vi "UDP Data Link - Configuration Utilities - Update Properties.vi"(6 "Tx?":bool, 8 "error in (no error)":errorcluster, 9 "Channel Paths":string[](array[string]), 10 "Channel Names":string[](array[string]), 11 "Item Ref in":T1 format="%.0x") -> (0 "error out":errorcluster, 3 "Item Ref out":T1=18446744073709551615 format="%.0x")   [LabVIEW 2015, in "UDP-Custom-Device System Explorer.lvlib"]
uses:
  UDP-Custom-Device System Explorer.lvlib
  <vilib>/NI Veristand/Custom Device API/Custom Device Item Ref.ctl
  Shared/Constants.vi
  <vilib>/NI Veristand/Custom Device API/Set Item Property (String Array).vi
  <vilib>/NI VeriStand/Custom Device API/Custom Device API.lvlib
  <vilib>/NI VeriStand/Custom Device Tools/Custom Device Utility Library/Custom Device Utility Library.lvlib
  Shared/UDP-Custom-Device Shared.lvlib
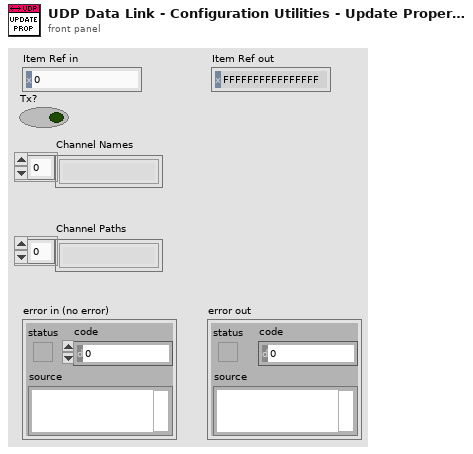
[diagram p1: front panel]
types:
  T1 = typedef "Custom Device API.lvlib/Custom Device Item Ref.ctl" = u64
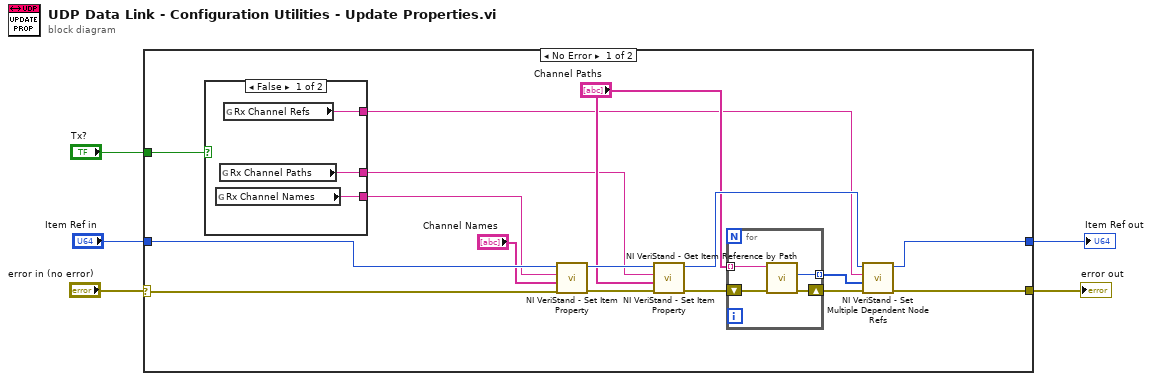
[diagram p0: block diagram]
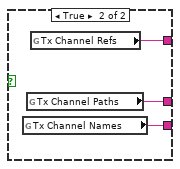
[diagram p2: hidden frame]
diagram:
  n1 = case shown="No Error" "error in (no error)" {
    selector: "error in (no error)" -> [w6 w33]
    tunnel: [w20 w33] -> w5
    tunnel: "Item Ref in" -> [w14 w32]
    tunnel: [w11 w32] -> w3
    tunnel: "Tx?" -> [w7 _]
    frame No Error {
      n2 = case shown="False" w7 {
        tunnel: [w24 w26] -> w10
        tunnel: [w23 w25] -> w9
        tunnel: [w22 w27] -> w8
        frame False {
          n3 = global read "Constants.vi" "Rx Channel Names"() -> (w24:string)
          n4 = global read "Constants.vi" "Rx Channel Paths"() -> (w23:string)
          n5 = global read "Constants.vi" "Rx Channel Refs"() -> (w22:string)
        }
        frame True {
          n6 = global read "Constants.vi" "Tx Channel Names"() -> (w26:string)
          n7 = global read "Constants.vi" "Tx Channel Paths"() -> (w25:string)
          n8 = global read "Constants.vi" "Tx Channel Refs"() -> (w27:string)
        }
      }
      n9 = call-poly <vilib>:"NI VeriStand - Set Item Property.vi"("error in (no error)"=w6, "Value"="Channel Names", "Property Name"=w10, "Item Ref in"=w14) -> ("error out"=w15:errorcluster, "Item Ref out"=w16:T1)  [unwired: 5 in, 1 out]
      n10 = call-poly <vilib>:"NI VeriStand - Set Item Property.vi"("error in (no error)"=w15, "Value"="Channel Paths", "Property Name"=w9, "Item Ref in"=w16) -> ("error out"=w19:errorcluster, "Item Ref out"=w18:T1)  [unwired: 5 in, 1 out]
      n11 = for {
        shift-right: [w30] -> w21
        shift-left: w19 -> [w31]
        tunnel: "Channel Paths" -> [w29] mode=indexing
        tunnel: [w28] -> w17 mode=indexing
        n12 = call <vilib>:"NI VeriStand - Get Item Reference by Path.vi"("error in (no error)"=w31, "Item Path in"=w29) -> ("error out"=w30:errorcluster, "Item Ref"=w28:T1)  [unwired: 6 in, 2 out]
      }
      n13 = call <vilib>:"NI VeriStand - Set Multiple Dependent Node Refs.vi"("error in (no error)"=w21, "Dependent Node Refs"=w17, "Base Property Name"=w8, "Item Ref in"=w18) -> ("error out"=w20:errorcluster, "Item Ref out"=w11:T1)  [unwired: 6 in]
    }
    frame Error {
    }
  }
  "error out" <- w5
  "Item Ref out" <- w3
